vi "LEBITplc.GetGUINames.vi"(0 "i ref in":refnum<vi>, 5 "error in (no error)":errorcluster) -> (14 "i ref out":refnum<vi>, 16 "GUINames":string[](array[string]), 19 "error out":errorcluster)   [LabVIEW 2014, in "LEBITplc.lvlib"]
uses:
  LEBITplc.lvlib
  CS_Core/BaseProcess/BaseProcess.lvlib
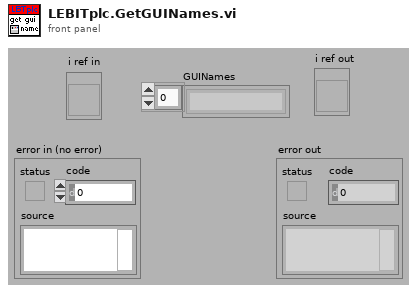
[diagram p1: front panel]
types:
  T1 = typedef "BaseProcess.lvlib/BaseProcess.i attribute.ctl" = cluster{"EventStatus":string, "EventError":i32, "PresetEvtWatchD":i32, "PresetPdcWatchD":i32, "EventTimeout":i32, "PeriodicInterval":i32, "Interface":string[], "Address":string[], "Special":string[], "PeriodicError":i32, "PeriodicStatus":string, "SuperProc":string, "Descriptors":T2[], "CaseRef":refnum<vi>, "PdcRef":refnum<vi>, "Thread Ref":refnum<vi>, "eventErrorID":i32, "eventStatusID":i32, "periodicErrorID":i32, "periodicStatusID":i32, "pdcCtrID":i32}
  T2 = typedef "BaseProcess.lvlib/BaseProcess.descriptor definition.ctl" = cluster{"selector":string, "descriptor":T3}
  T3 = typedef "BaseProcess.lvlib/BaseProcess.descriptor string definition.ctl" = string
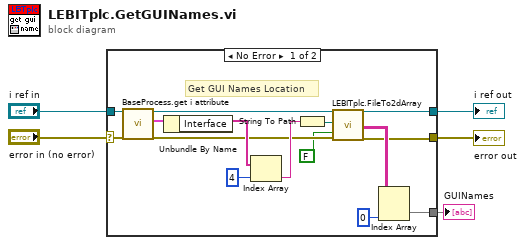
[diagram p0: block diagram]
diagram:
  n1 = case shown="No Error" "error in (no error)" {
    selector: "error in (no error)" -> [w14 w20]
    tunnel: "i ref in" -> [w19 w21]
    tunnel: [w7 w20] -> w2
    tunnel: [w18 w21] -> w4
    tunnel: [w9 _] -> w1
    frame No Error {
      # "Get GUI Names Location"
      n2 = call "BaseProcess.get i attribute.vi"("i ref in"=w19, "error in (no error)"=w14) -> ("i ref out"=w18:refnum<vi>, "i attribute"=w17:T1, "error out"=w8:errorcluster)  [unwired: 15 in]
      n3 = Unbundle By Name(w17) -> ("Interface"=w16:string[])
      n4 = Index Array(array=w16, index=4) -> (element=w13:string)
      n5 = String To Path(string=w13) -> (path=w12:path)
      n6 = call "LEBITplc.FileTo2dArray.vi"("file path (dialog if empty)"=w12, "Create if ness."=FALSE, "error in"=w8) -> ("Array"=w11:string[][], "error out"=w7:errorcluster)  [unwired: 15 in]
      n7 = Index Array(array=w11, index (col)=0 ("disabled index (col)")) -> (element=w9:string[])  [unwired: 1 in]
    }
    frame Error {
    }
  }
  "error out" <- w2
  "i ref out" <- w4
  "GUINames" <- w1
